vi "Initialize.vi"(5 "timeout, ms (300)":u32=300, 7 "address (1)":u8=1, 8 "error in (no error)":errorcluster, 10 "baud rate (19200)":u32=19200, 11 "port":refnum<visa-resource-name>) -> (0 "error out":errorcluster, 3 "RRG out":refnum<class "PL Eltochpribor RRG.lvclass">)   [LabVIEW 2015, in "PL Eltochpribor RRG.lvclass"]
doc: "Initializes connection to device using specified settings."
uses:
  PL Eltochpribor RRG.lvclass
  <vilib>/plasmapper/PL Modbus Client/PL Modbus Client.lvclass
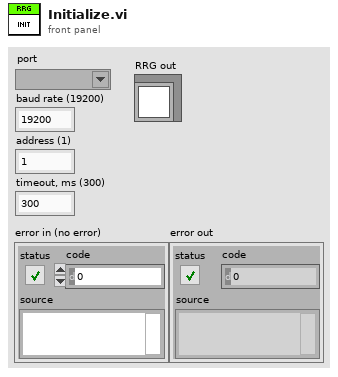
[diagram p1: front panel]
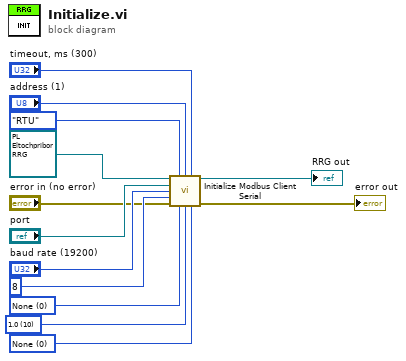
[diagram p0: block diagram]
diagram:
  w4 = u16 0 items=["None", "XON/XOFF", "RTS/CTS", "XON/XOFF & RTS/CTS", "DTR/DSR", "XON/XOFF & DTR/DSR"] ("flow control (none)")
  w5 = u16 10 items=["1.0"=10, "1.5"=15, "2.0"=20] ("stop bits (1.0)")
  w6 = u16 0 items=["None", "Odd", "Even", "Mark", "Space"] ("parity (even)")
  n1 = call <vilib>:"Initialize Modbus Client Serial.vi"("MODBUS in"=refnum<class "PL Eltochpribor RRG.lvclass"> refnum ("Eltochpribor RRG.lvclass"), "protocol (RTU)"=enum16{"RTU", "ASCII", "TCP"}."RTU", "station address (1)"="address (1)", "timeout, ms (300)"="timeout, ms (300)", "port"="port", "baud rate (9600)"="baud rate (19200)", "data bits (8)"=u16 8, "error in (no error)"="error in (no error)", "parity (even)"=w6, "stop bits (1.0)"=w5, "flow control (none)"=w4) -> ("MODBUS out"=→"RRG out":refnum<class "PL Eltochpribor RRG.lvclass">, "error out"=→"error out":errorcluster)  [unwired: 3 in]
